vi "Shutdown.vi"(8 "error in":errorcluster, 11 "Base Software in":refnum<class "Base Software.lvclass">) -> (0 "error out":errorcluster, 3 "Base Software out":refnum<class "Base Software.lvclass">)   [LabVIEW 2019, in "Base Software.lvlib" / "Main.lvlib" / "Base Software.lvclass"]
doc: "This routine transmits Stop Actor Messages for the instantiated Actors:\n\n1. <b>Fault Monitor</b>\n2. <b>Debugger</b>\n3. <b>Configuration UI</b>\n4. <b>Chronometer</b>\n5. <b>Manual UI</b>\n6. <b>Manual Buttons</b>\n7. <b>Report Generator</b>\n8. <b>Report Viewer</b>"
uses:
  Project/Base Software.lvclass
  Project/Base Software.lvclass/Base Software.ctl
  Custom Controls/Subordinate.ctl
  builds/Engine/Actor Framework.lvlibp/1abvi3w/vi.lib/ActorFramework/Message Enqueuer/Message Enqueuer.lvclass
  Custom Controls/Panel_Positions.ctl
  builds/Engine/Actor Framework.lvlibp/1abvi3w/vi.lib/ActorFramework/Stop Msg/Stop Msg.lvclass
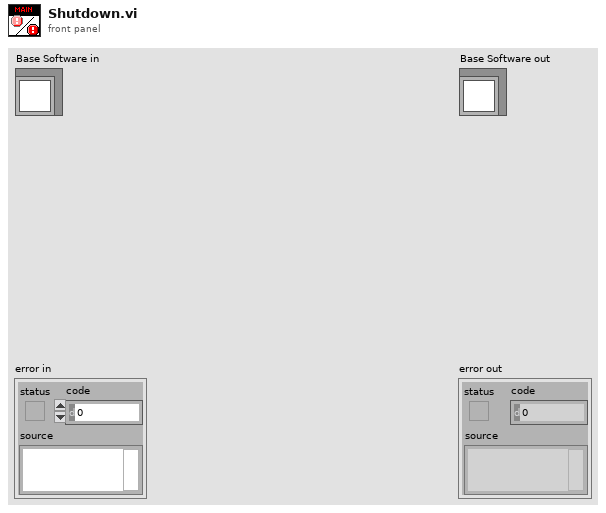
[diagram p1: front panel]
types:
  T1 = typedef "Base Software.lvlib/Main.lvlib/Base Software.lvclass/Subordinate.ctl" = cluster{"Identifier":string, "Enqueuer":refnum<class "Message Enqueuer.lvclass">, "Position":T2}
  T2 = typedef "Base Software.lvlib/Main.lvlib/Base Software.lvclass/Panel_Positions.ctl" = enum16{"Prime", "Right", "Bottom", "Left", "Mission"}
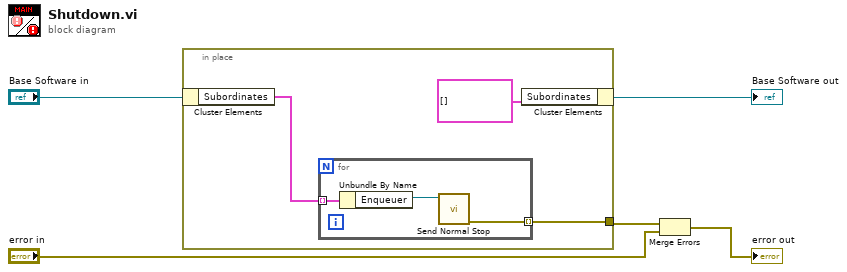
[diagram p0: block diagram]
diagram:
  n1 = in-place {
    in-place-border: [w6] -> w3
    n2 = in-place-cluster #1("Base Software in") -> ("Subordinates"=w7:T1[])
    n3 = for {
      tunnel: w7 -> [w11] mode=indexing
      tunnel: [w9] -> w6 mode=indexing
      n4 = Unbundle By Name(w11) -> ("Enqueuer"=w10:refnum<class "Message Enqueuer.lvclass">)
      n5 = call "Send Normal Stop.vi"("Message Enqueuer"=w10) -> ("error out"=w9:errorcluster)  [unwired: 10 in]
    }
    n6 = in-place-cluster #1("Subordinates"=T1[] []) -> (→"Base Software out":refnum<class "Base Software.lvclass">)
  }
  n7 = Merge Errors(w3, "error in") -> (→"error out":errorcluster)
